vi "Pi_Setup.vi"() -> ()   [LabVIEW 2022 SP3]
panel:
  in  "Tab Control":T1(tab)
  in  "password":string
  in  "SSID":string
  in  "Update SDCard":bool
  in  "wpa file":string="ctrl_interface=DIR=/var/run/wpa_supplicant GROUP=netdev\nupdate_config=1\ncountry=US\n\nnetwork={\n    ssid=\"<YOUR NETWORK NAME>\"\n    psk=\"<YOUR NETWORK PASSWORD>\"\n    key_mgmt=WPA-PSK\n}"
  # "Setting up the Pi headless"
  # "1. Making the SD Image"
  # "a. Get the burner from https://www.raspberrypi.org/software/ and make a standard image \nb. Mount the SD Card in your PC - and add enable_uart=1 to your config.txt text file\nc. Add start_x=1 to your config.txt text file to initialize the camera\nd. Create an empty file in the boot directory called ssh (this will initialize SSH on startup)\ne. Create a new file in the boot directory called wpa_supplicant.conf with this text in it (replace the all caps stuff with the correct settings)\nf. Eject the SD card and put it in the Pi and start it up\n\nNote: editing these files in TextEdit can add unwanted file extensions and hidden characters"
  # "https://learn.sparkfun.com/tutorials/headless-raspberry-pi-setup/serial-terminal"
  # "1. Connecting up"
  # "a. Load drivers for your machine https://www.adafruit.com/product/954\nb. Mac users, you might have to allow it in your System Preferences\nc. Connect the serial cable - Ground, Rx, and Tx\nd. Turn on the Pi - do you see code to your left?\ne. Get your IP Address\nf. turn on VNC (sudo raspi-config - and enable VNC)"
  # "2. Getting it on the WiFi"
  # "a. TuftsWireless and no password will only work if you have registered your Pi mac address on the Tufts portal already.  You can get your mac address by ifconfig in the terminal with the serial connection\n\nb. save the wpa_suplicant.conf file on the boot drive (the newly imaged SD Card on your PC) by clicking the button and then remove the card and put it into your rPi and start the Pi up.\n\nOR\n\nb. in the terminal - go to sudo nano /etc/wpa_supplicant/wpa_supplicant.conf and add it"
  # "3. Connecting over SSH"
  # "Setting up the Camera"
  # "a. connect up the ribbon cable (wires pointing away from USB ports)\n\nb."
  # "4. Chainging your password"
  # "From a command line prompt type passwd followed by the Enter key.\nType the current password followed by the Enter key.\nType the new password followed by the Enter key.\nRe-enter the new password followed by the Enter key.\nYour password has now been changed."
  # "https://github.com/PTC-Academic/SpatialToolbox-RaspberryPi"
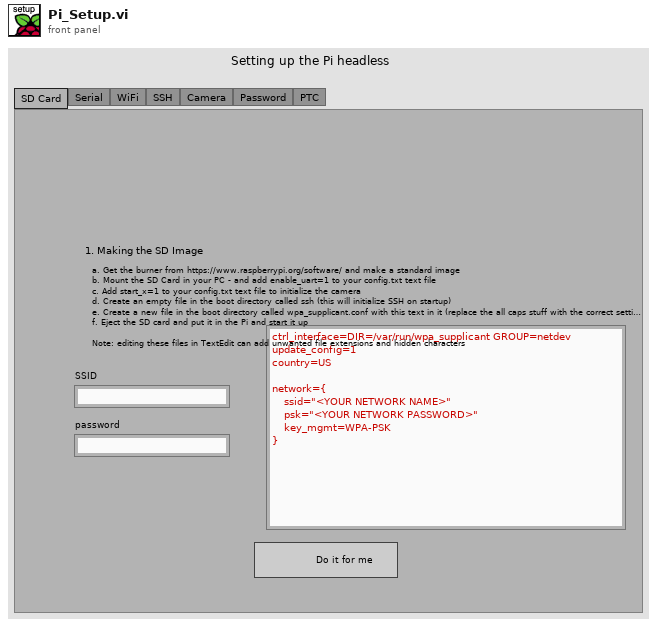
[diagram p1: front panel]
types:
  T1 = enum32{"SD Card", "Serial", "WiFi", "SSH", "Camera", "Password", "PTC"}
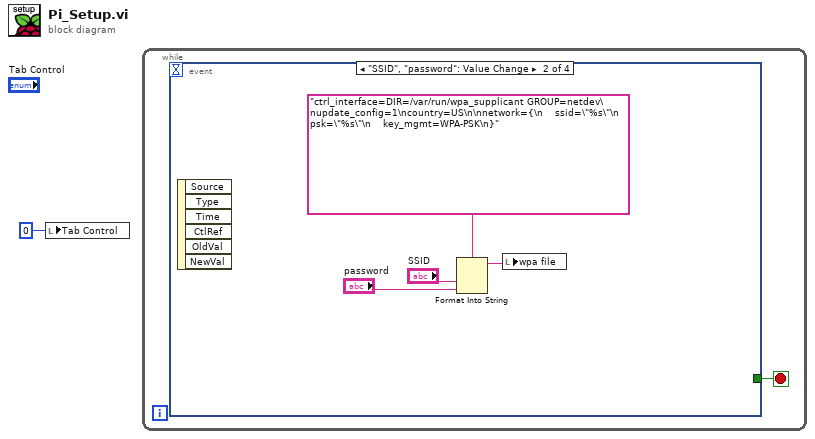
[diagram p0: block diagram]
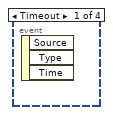
[diagram p2: hidden frame]
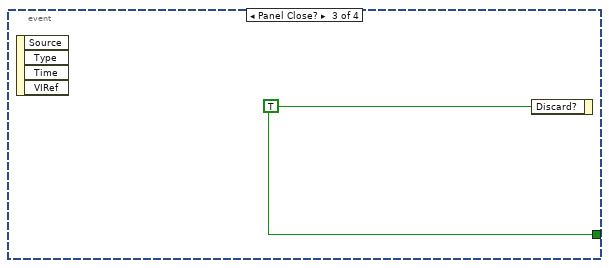
[diagram p3: hidden frame]
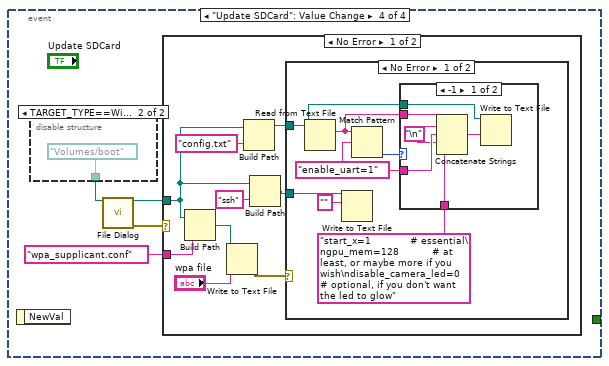
[diagram p4: hidden frame]
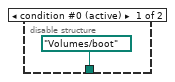
[diagram p5: hidden frame]
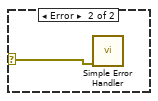
[diagram p7: hidden frame]
diagram:
  n1 = local write "Tab Control"(0) -> ()
  n2 = while {
    stop <- w2 stop-if-true
    n3 = event shown="[1] \"SSID\", \"password\": Value Change" {
      selector: _ -> [_ _ _ _]
      dyn-events: _ -> [_ _ _ _]
      timeout: _ -> [_ _ _ _]
      tunnel: [_ _ w7 _] -> w2
      event Timeout {
        n4 = event-data() -> ()  [unwired: 1 in, 3 out]
      }
      event "SSID", "password": Value Change {
        n5 = event-data() -> ()  [unwired: 1 in, 6 out]
        n6 = Format Into String(format string="ctrl_interface=DIR=/var/run/wpa_supplicant GROUP=netdev\nupdate_config=1\ncountry=US\n\nnetwork={\n    ssid=\"%s\"\n    psk=\"%s\"\n    key_mgmt=WPA-PSK\n}" ("wpa file"), "SSID", "password") -> (resulting string=w3:string)  [unwired: 2 in, 1 out]
        n7 = local write "wpa file"(w3) -> ()
      }
      event Panel Close? {
        w7 = TRUE ("Discard?")
        n8 = event-data() -> ()  [unwired: 1 in, 4 out]
        n9 = event-data("Discard?"=w7) -> ()  [unwired: 1 in, 1 out]
      }
      event "Update SDCard": Value Change {
        n10 = event-data() -> ()  [unwired: 1 in, 1 out]
        n11 = disable-structure shown="TARGET_TYPE==Windows" {
          disable-tunnel: [path "/Volumes/boot" ("start path") path "/Volumes/boot" ("start path")] -> w11
          frame condition #0 (active) {
          }
          frame condition #1 {
          }
        }
        n12 = call "File Dialog"("start path"=w11) -> ("selected path"=w9:path, "error out"=w10:errorcluster)  [unwired: 11 in, 2 out]
        n13 = case shown="No Error" w10 {
          tunnel: w9 -> [w15 _]
          tunnel: "wpa_supplicant.conf" ("default name") -> [w21 _]
          frame No Error {
            n14 = Build Path(base path=w15, name or relative path=w21) -> (appended path=w20:path)
            n15 = Write to Text File(file (use dialog)=w20, text="wpa file") -> (error out=w19:errorcluster)  [unwired: 2 in, 2 out]
            n16 = Build Path(base path=w15, name or relative path="config.txt" ("default name")) -> (appended path=w14:path)
            n17 = Build Path(base path=w15, name or relative path="ssh" ("default name")) -> (appended path=w17:path)
            n18 = case shown="No Error" w19 {
              selector: w19 -> [_ w36]
              tunnel: w17 -> [w29 _]
              tunnel: w14 -> [w25 _]
              frame No Error {
                w26 = "enable_uart=1" ("default name")
                n19 = Read from Text File(file (use dialog)=w25) -> (text=w27:string)  [unwired: 3 in, 3 out]
                n20 = Write to Text File(file (use dialog)=w29, text="") -> ()  [unwired: 2 in, 3 out]
                n21 = Match Pattern(string=w27, regular expression=w26) -> (offset past match=w28:i32)  [unwired: 1 in, 3 out]
                n22 = case shown="-1" w28 {
                  tunnel: w27 -> [w35 _]
                  tunnel: w26 -> [w34 _]
                  tunnel: w25 -> [w32 _]
                  tunnel: "start_x=1             # essential\ngpu_mem=128           # at least, or maybe more if you wish\ndisable_camera_led=0  # optional, if you don't want the led to glow" ("default name") -> [w30 _]
                  frame -1 {
                    w31 = "\n"
                    n23 = Concatenate Strings(w35, w31, w34, w31, w30) -> (w33:string)
                    n24 = Write to Text File(file (use dialog)=w32, text=w33) -> ()  [unwired: 2 in, 3 out]
                  }
                  frame Default {
                  }
                }
              }
              frame Error {
                n25 = call <vilib>:"Simple Error Handler.vi"("error in (no error)"=w36) -> ()  [unwired: 4 in, 5 out]
              }
            }
          }
          frame Error {
          }
        }
      }
    }
  }
